vi "GetDriverName.vi"(8 "Error In":errorcluster, 11 "reference in":refnum<class "VdDigitalControl_Simulated.lvclass">) -> (0 "Error Out":errorcluster, 2 "DriverName":string, 3 "reference out":refnum<class "VdDigitalControl_Simulated.lvclass">)   [LabVIEW 2020, in "VdDigitalControl_Simulated.lvclass"]
uses:
  VdDigitalControl_Simulated.lvclass
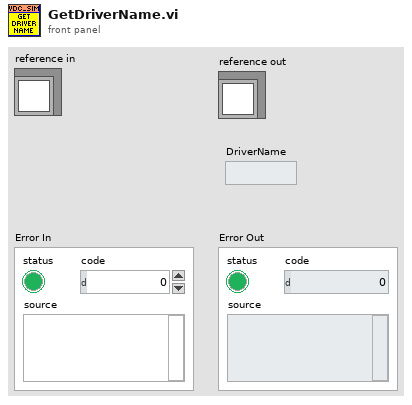
[diagram p1: front panel]
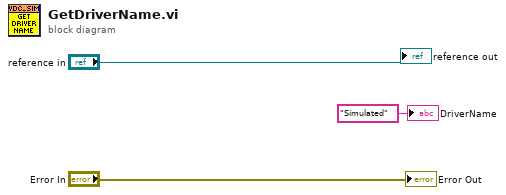
[diagram p0: block diagram]
diagram:
  "Error Out" <- "Error In"
  "reference out" <- "reference in"
  "DriverName" <- "Simulated" ("DriverName")
